vi "Sonde Measurement Array to Cluster.vi"(10 "Measurements In":dbl[](array[numeric])) -> (2 "Battery Voltage (V)":dbl, 3 "Cluster Out":T1 caption="Cluster")   [LabVIEW 2016]
uses:
  activeXtest/activeXtest 2015 Folder/sonde cluster.ctl
panel:
  in  "Cluster In":T1 caption="Cluster"
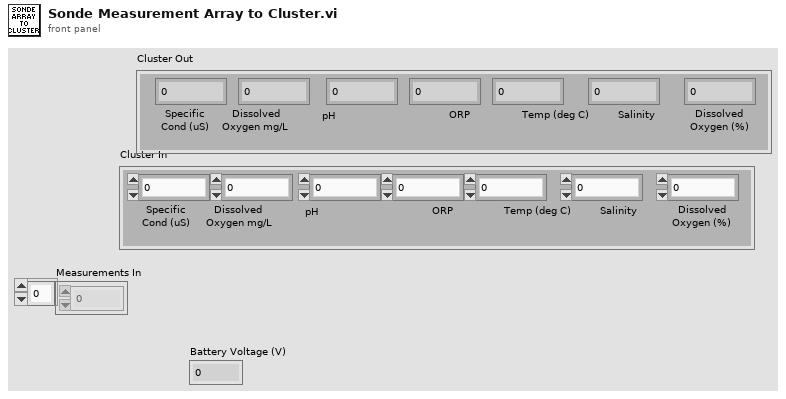
[diagram p1: front panel]
types:
  T1 = typedef "sonde cluster.ctl" = cluster{"Specific\nCond (uS)":dbl, "Dissolved\nOxygen mg/L":dbl, "pH":dbl, "ORP":dbl, "Temp (deg C)":dbl, "Salinity":dbl, "Dissolved\nOxygen (%)":dbl}
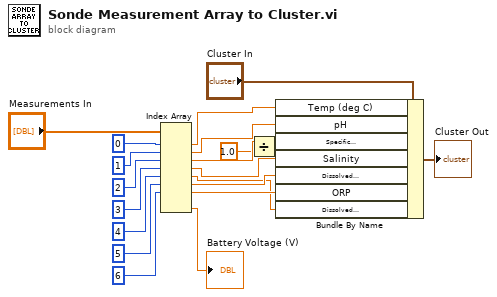
[diagram p0: block diagram]
diagram:
  n1 = Index Array(array="Measurements In", index #1=0 ("index"), index #2=1 ("index"), index #3=2 ("index"), index #4=3 ("index"), index #5=4 ("index"), index #6=5 ("index"), index #7=6 ("index")) -> (element #1=w7:dbl, element #2=w11:dbl, element #3=w12:dbl, element #4=w17:dbl, element #5=w3:dbl, element #6=w18:dbl, element #7=w19:dbl, element #9=→"Battery Voltage (V)":dbl)  [unwired: 2 in, 1 out]
  n2 = Divide(x=w12, y=1.0) -> (x/y=w2:dbl)
  n3 = Bundle By Name(cluster="Cluster In", "Temp (deg C)"=w7, "pH"=w11, "Specific\nCond (uS)"=w2, "Salinity"=w17, "Dissolved\nOxygen mg/L"=w18, "ORP"=w19, "Dissolved\nOxygen (%)"=w3) -> (→"Cluster Out":T1)
